vi "Handle Drop.vi"(4 "Mods":cluster{"Double Click":bool, "Menu Key":bool}, 5 "Tag":string, 6 "PlatMods":T2, 7 "Button":u16, 8 "error in (no error)":errorcluster, 9 "Coords":T1, 10 "Available Data Names":string[](array[string]), 11 "Process Builder View in":refnum<class "Process Builder View.lvclass">) -> (0 "error out":errorcluster, 2 "Discard?":bool, 3 "Process Builder View out":refnum<class "Process Builder View.lvclass">)   [LabVIEW 2019, in "Process Builder View.lvclass"]
uses:
  <vilib>/gpm_packages/@cs/Car-wash/Source/Process Builder View/Process Builder View.lvclass
  C:/Program Files/National Instruments/LabVIEW 2019/vi.lib/gpm_packages/@cs/Test-executive-builder/Source/Test Executive Builder View/Test Executive Builder View/Test Executive Builder View.lvclass
  <vilib>/Utility/miscctls.llb/LVPoint32TypeDef.ctl
  <vilib>/gpm_packages/@cs/Test-executive-builder/Source/Test Executive Builder View/Test Executive Builder View/Test Executive Builder View.lvclass/Test Executive Builder View.ctl
  <vilib>/gpm_packages/@cs/Test-executive-builder/Source/Application Dependencies/Drop Element.ctl
  <vilib>/gpm_packages/@cs/Test-executive-builder/Source/Test Executive Builder View/Tree Click Interpreter/Tree Click Interpreter.lvclass
  <vilib>/gpm_packages/@cs/Test-executive-builder/Source/Test Executive Builder View/Test Executive Builder View/Test Executive Builder View.lvclass
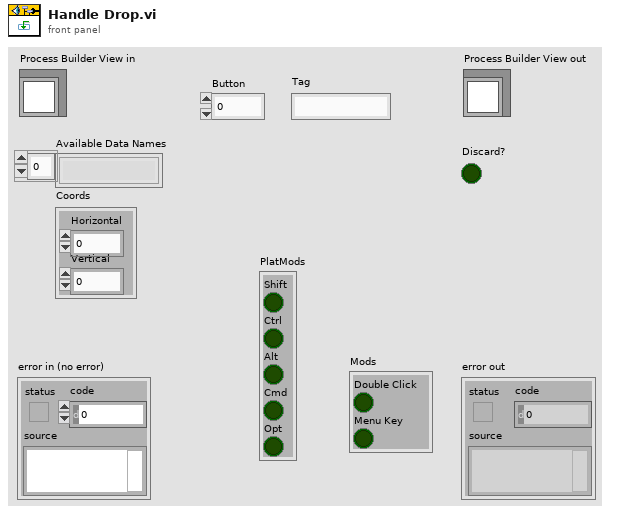
[diagram p1: front panel]
types:
  T1 = typedef "LVPoint32TypeDef.ctl" = cluster{"Horizontal":i32, "Vertical":i32}
  T2 = cluster{"Shift":bool, "Ctrl":bool, "Alt":bool, "Cmd":bool, "Opt":bool}
  T3 = typedef "Drop Element.ctl" = cluster{"Parent ID":string, "Insertion Index":i32, "Tag":string, "Ctrl":bool}
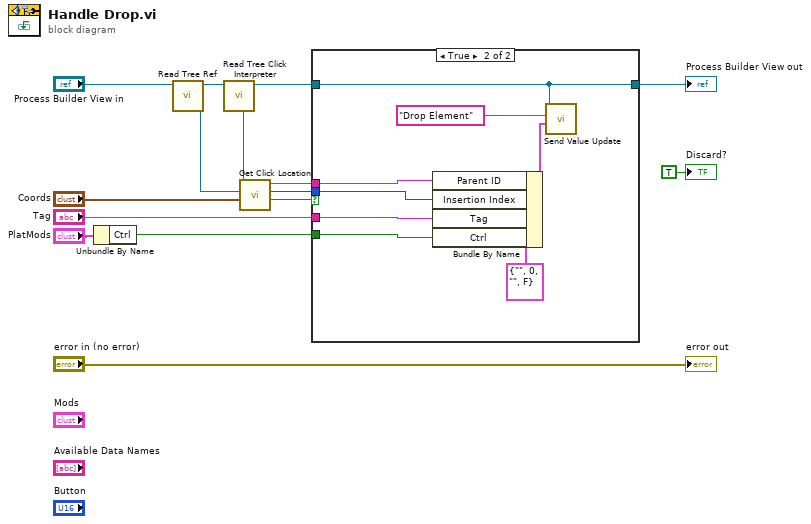
[diagram p0: block diagram]
diagram:
  n1 = Unbundle By Name("PlatMods") -> ("Ctrl"=w8:bool)
  n2 = call <vilib>:"Read Tree Ref.vi"("Test Executive Builder View in"="Process Builder View in") -> ("Tree Ref"=w11:refnum<vi>, "Test Executive Builder View out"=w14:refnum<class "Process Builder View.lvclass">)  [unwired: 9 in]
  n3 = call <vilib>:"Read Tree Click Interpreter.vi"("Test Executive Builder View in"=w14) -> ("Test Executive Builder View out"=w13:refnum<class "Process Builder View.lvclass">, "Tree Click Interpreter"=w12:refnum<class "Tree Click Interpreter.lvclass">)  [unwired: 9 in]
  n4 = call-dynamic "Get Click Location.vi"("Coords"="Coords", "Tree Refnum"=w11, "Tree Click Interpreter in"=w12) -> ("Valid?"=w7:bool, "Insertion Index"=w9:i32, "Parent ID"=w10:string)  [unwired: 4 in, 2 out]
  n5 = case shown="True" w7 {
    tunnel: w13 -> [w16 w18]
    tunnel: w10 -> [_ w22]
    tunnel: w9 -> [_ w21]
    tunnel: "Tag" -> [_ w20]
    tunnel: w8 -> [_ w19]
    tunnel: [w16 w18] -> w5
    frame False {
    }
    frame True {
      n6 = Bundle By Name(cluster=T3 {"Parent ID"="", "Insertion Index"=0, "Tag"="", "Ctrl"=FALSE} ("Drop Element"), "Parent ID"=w22, "Insertion Index"=w21, "Tag"=w20, "Ctrl"=w19) -> (w17:T3)
      n7 = call-dynamic "Send Value Update.vi"("Value"=w17, "Datum Name"="Drop Element", "IViewable in"=w18) -> ()  [unwired: 8 in, 1 out]
    }
  }
  "Process Builder View out" <- w5
  "error out" <- "error in (no error)"
  "Discard?" <- TRUE ("Discard?")
